vi "Write Page ActionVI Properties.vi"(8 "Error In":errorcluster, 10 "ActionVIs Properties":T1, 11 "Custom Device Page .NET Ref In":refnum<k24>) -> (0 "Error Out":errorcluster, 3 "Custom Device Page .NET Ref Out":refnum<k24>)   [LabVIEW 2019, in "VeriStand Custom Device XML Parser.lvlib"]
doc: "Sets the properties of each action VI"
uses:
  VeriStand Custom Device XML Parser.lvlib
  NationalInstruments.VeriStand.XMLReader
  XML Controls/ActionVIs Properties.ctl
  XML Controls/Path Cluster.ctl
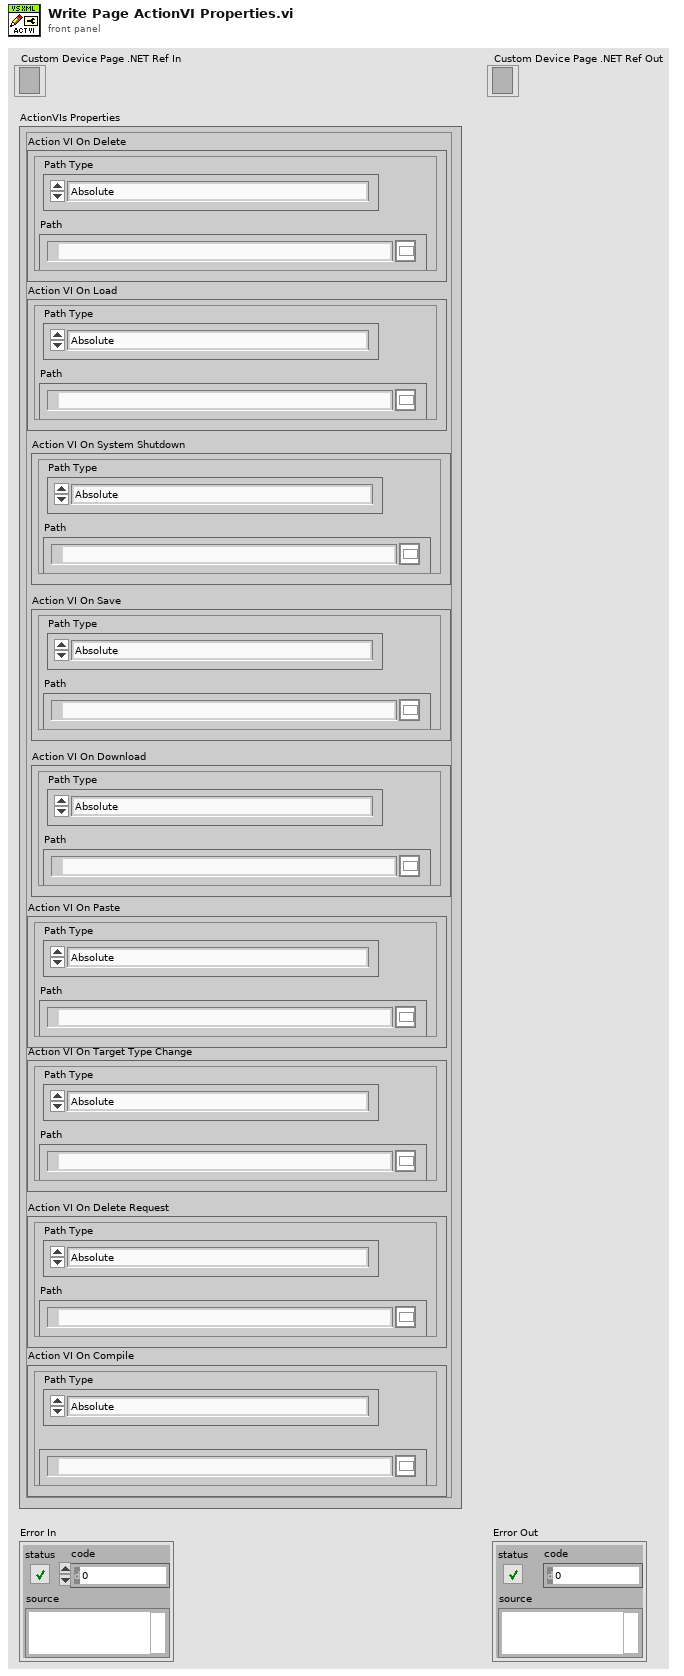
[diagram p1: front panel]
types:
  T1 = typedef "VeriStand Custom Device XML Parser.lvlib/ActionVIs Properties.ctl" = cluster{"Action VI On Delete":T2, "Action VI On Load":T2, "Action VI On Paste":T2, "Action VI On Target Type Change":T2, "Action VI On Delete Request":T2, "Action VI On Compile":T2, "Action VI On System Shutdown":T2, "Action VI On Save":T2, "Action VI On Download":T2}
  T2 = typedef "VeriStand Custom Device XML Parser.lvlib/Path Cluster.ctl" = cluster{"Path":path, "Path Type":enum16{"Absolute", "To Base", "To Common Doc Dir", "To Application Data Dir"}}
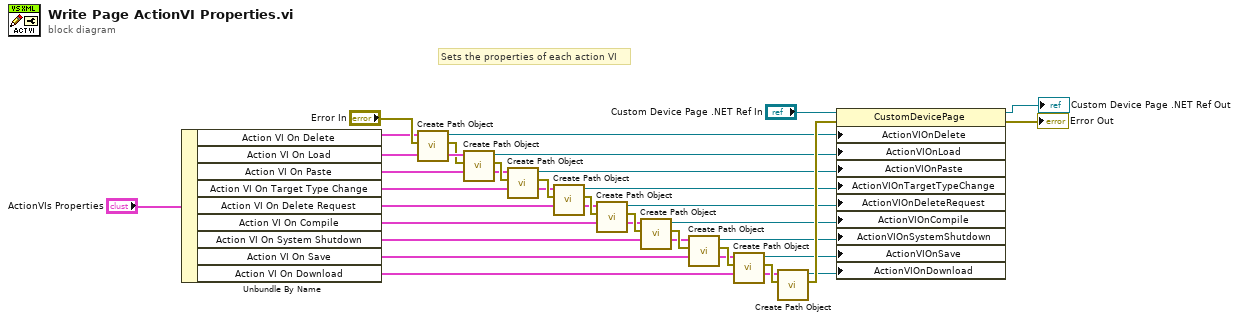
[diagram p0: block diagram]
diagram:
  # "Sets the properties of each action VI"
  n1 = Unbundle By Name("ActionVIs Properties") -> ("Action VI On Delete"=w3:T2, "Action VI On Load"=w7:T2, "Action VI On Paste"=w9:T2, "Action VI On Target Type Change"=w12:T2, "Action VI On Delete Request"=w14:T2, "Action VI On Compile"=w16:T2, "Action VI On System Shutdown"=w17:T2, "Action VI On Save"=w18:T2, "Action VI On Download"=w19:T2)
  n2 = call "Create Path Object.vi"("Error In"="Error In", "Path Data Cluster"=w3) -> ("Error Out"=w6:errorcluster, "Path .NET Ref"=w5:refnum<k24>)  [unwired: 8 in]
  n3 = call "Create Path Object.vi"("Error In"=w6, "Path Data Cluster"=w7) -> ("Error Out"=w10:errorcluster, "Path .NET Ref"=w8:refnum<k24>)  [unwired: 8 in]
  n4 = call "Create Path Object.vi"("Error In"=w10, "Path Data Cluster"=w9) -> ("Error Out"=w13:errorcluster, "Path .NET Ref"=w11:refnum<k24>)  [unwired: 8 in]
  n5 = call "Create Path Object.vi"("Error In"=w13, "Path Data Cluster"=w12) -> ("Error Out"=w15:errorcluster, "Path .NET Ref"=w24:refnum<k24>)  [unwired: 8 in]
  n6 = call "Create Path Object.vi"("Error In"=w15, "Path Data Cluster"=w14) -> ("Error Out"=w20:errorcluster, "Path .NET Ref"=w25:refnum<k24>)  [unwired: 8 in]
  n7 = call "Create Path Object.vi"("Error In"=w20, "Path Data Cluster"=w16) -> ("Error Out"=w21:errorcluster, "Path .NET Ref"=w26:refnum<k24>)  [unwired: 8 in]
  n8 = call "Create Path Object.vi"("Error In"=w21, "Path Data Cluster"=w17) -> ("Error Out"=w22:errorcluster, "Path .NET Ref"=w27:refnum<k24>)  [unwired: 8 in]
  n9 = call "Create Path Object.vi"("Error In"=w22, "Path Data Cluster"=w18) -> ("Error Out"=w23:errorcluster, "Path .NET Ref"=w28:refnum<k24>)  [unwired: 8 in]
  n10 = call "Create Path Object.vi"("Error In"=w23, "Path Data Cluster"=w19) -> ("Error Out"=w30:errorcluster, "Path .NET Ref"=w29:refnum<k24>)  [unwired: 8 in]
  n11 = property class="CustomDevicePage"(reference="Custom Device Page .NET Ref In", error in=w30, "ActionVIOnDelete"=w5, "ActionVIOnLoad"=w8, "ActionVIOnPaste"=w11, "ActionVIOnTargetTypeChange"=w24, "ActionVIOnDeleteRequest"=w25, "ActionVIOnCompile"=w26, "ActionVIOnSystemShutdown"=w27, "ActionVIOnSave"=w28, "ActionVIOnDownload"=w29) -> (reference out=→"Custom Device Page .NET Ref Out":refnum<k24>, error out=→"Error Out":errorcluster)
